vi "Test MFC Init.vi"   [LabVIEW 2012]
uses:
  <userlib>/Serialization/Formatter/Formatter.lvclass
  cPAS.lvclass
types:
  T1 = enum16{"No paths embedded", "One path with each object", "All paths with top object"}
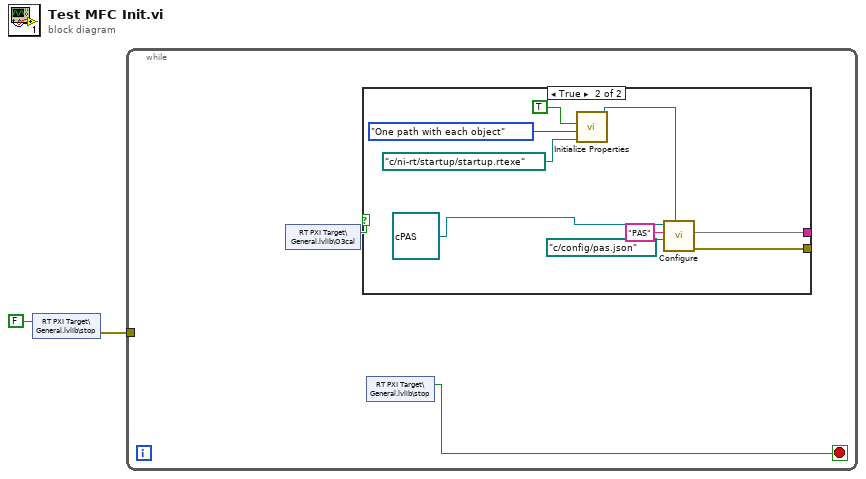
[diagram p0: block diagram]
diagram:
  n1 = shared-variable "RT PXI Target\\General.lvlib\\stop"(FALSE ("stop")) -> (error out=w1:errorcluster)  [unwired: 1 in]
  n2 = while {
    tunnel: w1 -> [_]
    stop <- w4 stop-if-true
    n3 = shared-variable "RT PXI Target\\General.lvlib\\O3cal"() -> (w3:bool)  [unwired: 1 in, 1 out]
    n4 = case shown="True" w3 {
      tunnel: [_ w6] -> _
      tunnel: [_ w5] -> _
      frame False {
      }
      frame True {
        n5 = call <userlib>:"Initialize Properties.vi"("Absolute Path For Dynamic Loading"=path "c:/ni-rt/startup/startup.rtexe", "Path Embedding"=T1."One path with each object", "Include all fields?"=TRUE) -> ("Formatter out"=w11:refnum<class "Formatter.lvclass">)  [unwired: 8 in]
        n6 = call-dynamic "Configure.vi"(7:w11, 9:path "c:/config/pas.json" ("file path"), "name"="PAS", "PAS in"=refnum<class "cPAS.lvclass"> refnum ("cPAS")) -> ("error out"=w5:errorcluster, 2:w6)  [unwired: 5 in, 1 out]
      }
    }
    n7 = shared-variable "RT PXI Target\\General.lvlib\\stop"() -> (w4:bool)  [unwired: 1 in, 1 out]
  }
